vi "全局变量接收数据(subvi).vi"() -> ()   [LabVIEW 2010]
uses:
  传递波形全局变量.vi
panel:
  out "延时":u32
  out "波形图表":dbl(graph)
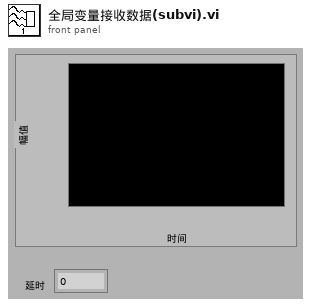
[diagram p1: front panel]
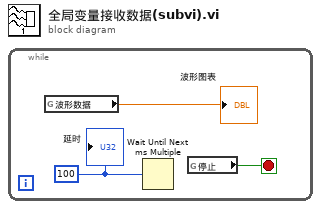
[diagram p0: block diagram]
diagram:
  n1 = while {
    stop <- w3 stop-if-true
    w1 = u32 100 ("millisecond multiple")
    n2 = global read "传递波形全局变量.vi" "波形数据"() -> (→"波形图表":dbl)
    n3 = Wait Until Next ms Multiple(millisecond multiple=w1) -> ()  [unwired: 1 out]
    n4 = global read "传递波形全局变量.vi" "停止"() -> (w3:bool)
    "延时" <- w1
  }
